vi "scp.vi"(6 "remote path":string, 7 "File":T1, 8 "error in (no error)":errorcluster, 10 "Console In":string, 11 "Python in":cluster{"Python":refnum<k35>, "py file":path}) -> (0 "error out":errorcluster, 2 "Console Out":string, 3 "Python out":cluster{"Python":refnum<k35>, "py file":path})   [LabVIEW 2020]
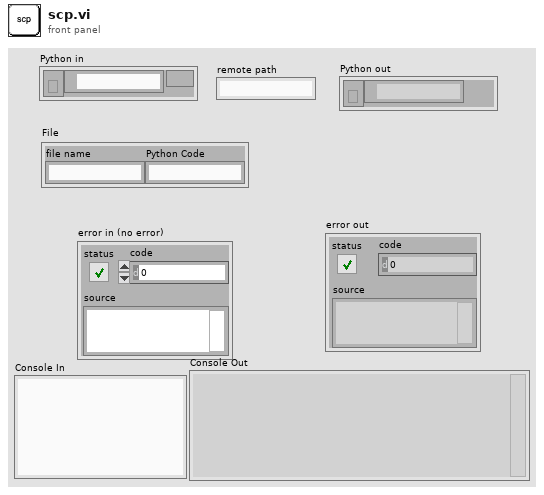
[diagram p1: front panel]
types:
  T1 = cluster{"file name":string, "Python Code":string}
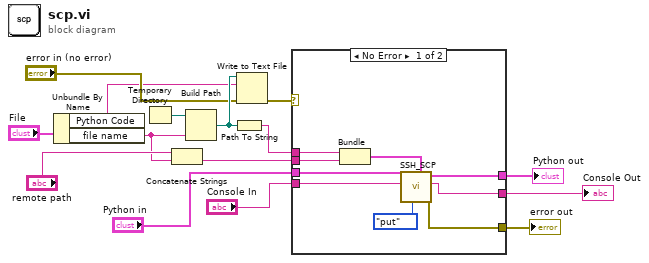
[diagram p0: block diagram]
diagram:
  n1 = Unbundle By Name("File") -> ("Python Code"=w5:string, "file name"=w1:string)
  n2 = Temporary Directory() -> (w4:path)
  n3 = Concatenate Strings("remote path", w1) -> (w3:string)
  n4 = Build Path(base path=w4, name or relative path=w1) -> (appended path=w15:path)
  n5 = Path To String(path=w15) -> (string=w14:string)
  n6 = Write to Text File(file (use dialog)=w15, text=w5, error in="error in (no error)") -> (error out=w12:errorcluster)  [unwired: 1 in, 2 out]
  n7 = case shown="No Error" w12 {
    selector: w12 -> [_ w27]
    tunnel: w14 -> [w24 _]
    tunnel: w3 -> [w23 _]
    tunnel: [w20 w26] -> w11
    tunnel: "Python in" -> [w19 w26]
    tunnel: [w18 w27] -> w9
    tunnel: [w17 w25] -> w8
    tunnel: "Console In" -> [w16 w25]
    frame No Error {
      n8 = Bundle(w24, w23) -> (w21:cluster{string, string})  [unwired: 1 in]
      n9 = call "SSH_SCP.vi"("Task"=enum16{"put", "get", "put folder"}."put", "scp"=w21, "Console In"=w16, "Python in"=w19) -> ("error out"=w18:errorcluster, "Console Out"=w17:string, "Python out"=w20:cluster{"Python":refnum<k35>, "py file":path})  [unwired: 5 in]
    }
    frame Error {
    }
  }
  "error out" <- w9
  "Python out" <- w11
  "Console Out" <- w8
